vi "CameraInit.vi"(0 "folder path":path, 1 "start time":timestamp, 2 "error in (no error)":errorcluster) -> (3 "error out":errorcluster, 4 "Color AVI out":T2, 5 "Color session out":T1, 6 "BW AVI out":T2, 7 "BW Session Out":T1)   [LabVIEW 2020]
uses:
  <vilib>/vision/Avi.llb/IMAQ AVI2 Refnum.ctl
  <vilib>/userdefined/High Color/IMAQdx.ctl
  <vilib>/vision/driver/NI_Vision_Acquisition_Software.lvlib
  <resource>/objmgr/imaqdx.rc
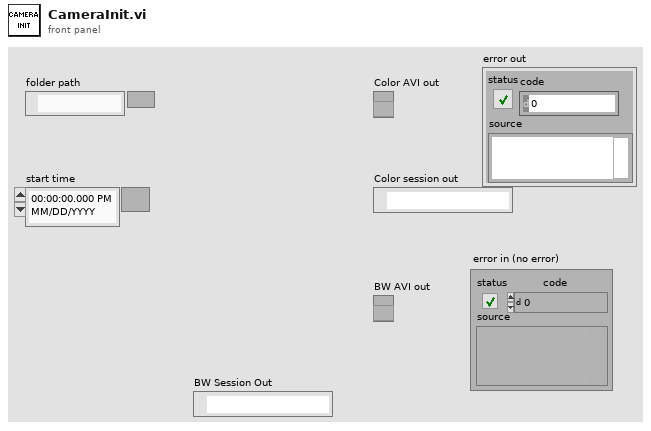
[diagram p1: front panel]
types:
  T1 = typedef "IMAQdx.ctl" = refnum<k21>
  T2 = typedef "IMAQ AVI2 Refnum.ctl" = refnum<k20>
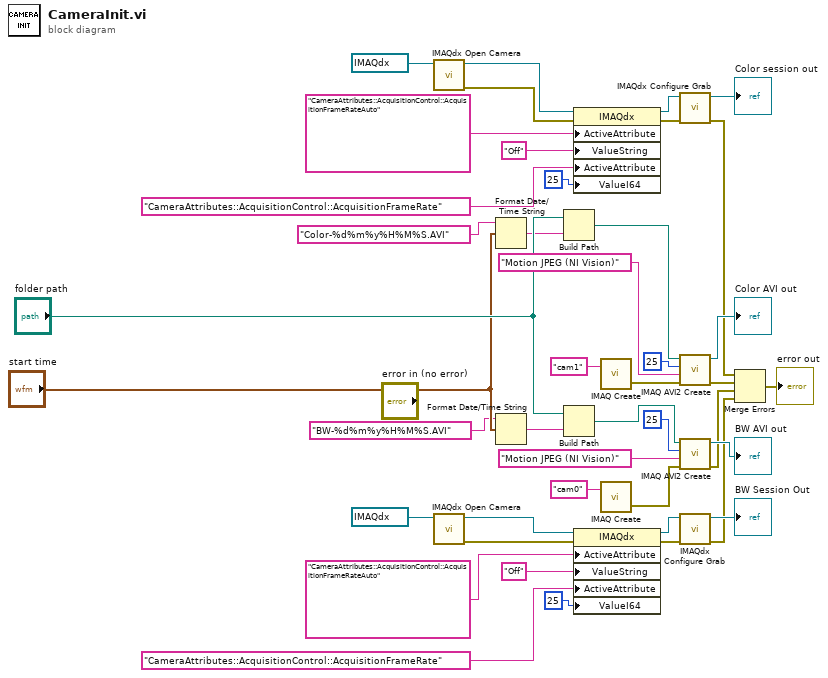
[diagram p0: block diagram]
diagram:
  n1 = call <vilib>:"IMAQdx Open Camera.vi"("Session In"=T1 "cam0") -> ("error out"=w18:errorcluster, "Session Out"=w16:T1)  [unwired: 9 in]
  n2 = call <vilib>:"IMAQdx Open Camera.vi"("Session In"=T1 "cam1") -> ("error out"=w9:errorcluster, "Session Out"=w7:T1)  [unwired: 9 in]
  n3 = Format Date/Time String(time format string (%c)="Color-%d%m%y%H%M%S.AVI", seconds (now)="start time") -> (date/time string=w32:string)  [unwired: 1 in]
  n4 = Format Date/Time String(time format string (%c)="BW-%d%m%y%H%M%S.AVI", seconds (now)="start time") -> (date/time string=w29:string)  [unwired: 1 in]
  n5 = Build Path(base path="folder path", name or relative path=w32) -> (appended path=w33:path)
  n6 = Build Path(base path="folder path", name or relative path=w29) -> (appended path=w30:path)
  n7 = property class="IMAQdx"(reference=w16, error in=w18, "ActiveAttribute"="CameraAttributes::AcquisitionControl::AcquisitionFrameRateAuto", "ValueString"="Off", "ActiveAttribute"="CameraAttributes::AcquisitionControl::AcquisitionFrameRate", "ValueI64"=u32 25 ("ValueU32")) -> (reference out=w17:T1, error out=w19:errorcluster)
  n8 = property class="IMAQdx"(reference=w7, error in=w9, "ActiveAttribute"="CameraAttributes::AcquisitionControl::AcquisitionFrameRateAuto", "ValueString"="Off", "ActiveAttribute"="CameraAttributes::AcquisitionControl::AcquisitionFrameRate", "ValueI64"=u32 25 ("ValueU32")) -> (reference out=w8:T1, error out=w10:errorcluster)
  n9 = call "IMAQ Create"("Image Name"="cam1") -> ("error out"=w25:errorcluster)  [unwired: 4 in, 1 out]
  n10 = call "IMAQ Create"("Image Name"="cam0") -> ("error out"=w26:errorcluster)  [unwired: 4 in, 1 out]
  n11 = call <vilib>:"IMAQdx Configure Grab.vi"("error in"=w19, "Session In"=w17) -> ("error out"=w5:errorcluster, "Session Out"=→"Color session out":T1)  [unwired: 8 in]
  n12 = call "IMAQ AVI2 Create"("error in (no error)"=w25, "Codec"="Motion JPEG (NI Vision)", "Frames Per Second"=u32 25, "AVI Path"=w33) -> ("error out"=w4:errorcluster, "AVI Refnum"=→"Color AVI out":T2)  [unwired: 6 in]
  n13 = call "IMAQ AVI2 Create"("error in (no error)"=w26, "Codec"="Motion JPEG (NI Vision)", "Frames Per Second"=u32 25, "AVI Path"=w30) -> ("error out"=w3:errorcluster, "AVI Refnum"=→"BW AVI out":T2)  [unwired: 6 in]
  n14 = call <vilib>:"IMAQdx Configure Grab.vi"("error in"=w10, "Session In"=w8) -> ("error out"=w2:errorcluster, "Session Out"=→"BW Session Out":T1)  [unwired: 8 in]
  n15 = Merge Errors(w5, w4, w3, w2) -> (→"error out":errorcluster)
